vi "subSetSourcePath.vi"(7 "Project path":path, 8 "error in (no error)":errorcluster, 9 "ProjectItem path":path, 10 "Name":string, 11 "SolutionBuilder in":refnum<class "SolutionBuilder.lvclass">) -> (0 "error out":errorcluster, 3 "SolutionBuilder out":refnum<class "SolutionBuilder.lvclass">)   [LabVIEW 2020, in "SolutionBuilder.lvlib" / "SolutionBuilder.lvclass"]
uses:
  SolutionBuilder.lvclass
  SolutionBuilder.lvclass/SolutionBuilder.ctl
  ProjectItem/ProjectItem.lvclass
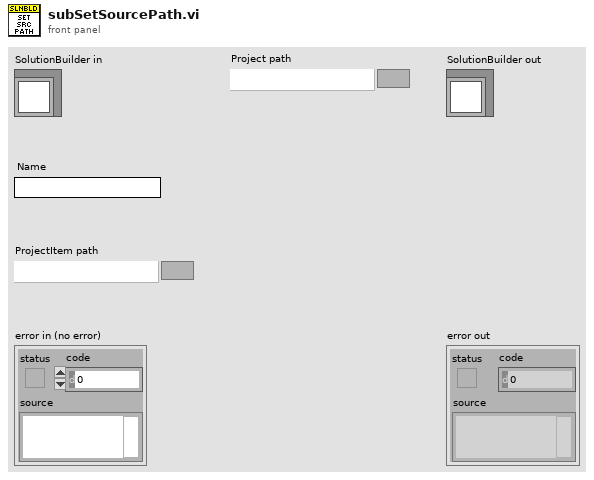
[diagram p1: front panel]
types:
  T1 = typedef "SolutionBuilder.lvlib/SolutionBuilder.lvclass/ProjectItemMap.ctl" = map{path, refnum<class "ProjectItem.lvclass">[]}
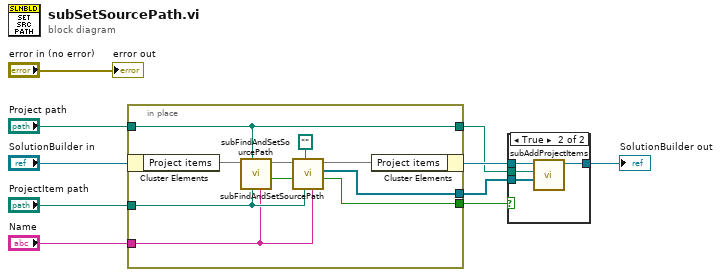
[diagram p0: block diagram]
diagram:
  n1 = in-place {
    in-place-border: "Project path" -> [w16]
    in-place-border: "Name" -> [w11]
    in-place-border: "ProjectItem path" -> [w12]
    in-place-border: [w19] -> w5
    in-place-border: [w13] -> w3
    in-place-border: [w16] -> w1
    n2 = in-place-cluster #1("SolutionBuilder in") -> ("Project items"=w18:T1)
    n3 = call "subFindAndSetSourcePath.vi"("Name"=w11, "ProjectItem path"=w12, "Owning project"=w16, "Project items in"=w18) -> ("Found"=w14:bool, "Project items out"=w17:T1)  [unwired: 5 in, 1 out]
    n4 = call "subFindAndSetSourcePath.vi"("Name"=w11, "ProjectItem path"=w12, "Owning project"=path "", "Skip"=w14, "Project items in"=w17) -> ("Found"=w13:bool, "Item found"=w19:refnum<class "ProjectItem.lvclass">[], "Project items out"=w20:T1)  [unwired: 4 in]
    n5 = in-place-cluster #1("Project items"=w20) -> (w7:refnum<class "SolutionBuilder.lvclass">)
  }
  n6 = case shown="True" w3 {
    tunnel: w7 -> [w21 w25]
    tunnel: [w21 w24] -> w6
    tunnel: w5 -> [_ w23]
    tunnel: w1 -> [_ w22]
    frame False {
    }
    frame True {
      n7 = call "subAddProjectItems.vi"("ProjectItems"=w23, "Owning project"=w22, "SolutionBuilder in"=w25) -> ("SolutionBuilder out"=w24:refnum<class "SolutionBuilder.lvclass">)  [unwired: 7 in, 1 out]
    }
  }
  "SolutionBuilder out" <- w6
  "error out" <- "error in (no error)"
